vi "CANTest2.vi"() -> ()   [LabVIEW 2009]
uses:
  <vilib>/Platform/TimedLoop/XDataNode/XDataNode.xnode
  <vilib>/Platform/TimedLoop/XDataNode/loadlvalarms.vi
  <vilib>/Platform/TimedLoop/XDataNode/timing_clust.ctl
  <vilib>/Platform/TimedLoop/XDataNode/nitl_modes.ctl
  <vilib>/Platform/TimedLoop/XDataNode/wakeup.ctl
  <vilib>/Platform/TimedLoop/XDataNode/XDNodeRunTimeDep.lvlib
  CAN.lvlib
  Serial.lvlib
  CAN/SubVIs/CAN Jaguar Control Mode.ctl
panel:
  out "read buffer":u8[](array[numeric])
  out "is Timeout":bool
  out "is Corrupted":bool
  out "read data":u8[](array[numeric]) format="%.0x"
  in  "data":u8[](array[numeric]) format="%.0x"
  in  "messageID":u32 format="%.0x"
  out "error out":errorcluster
  in  "OK Button":bool
  in  "stop 2":bool
  in  "stop":bool
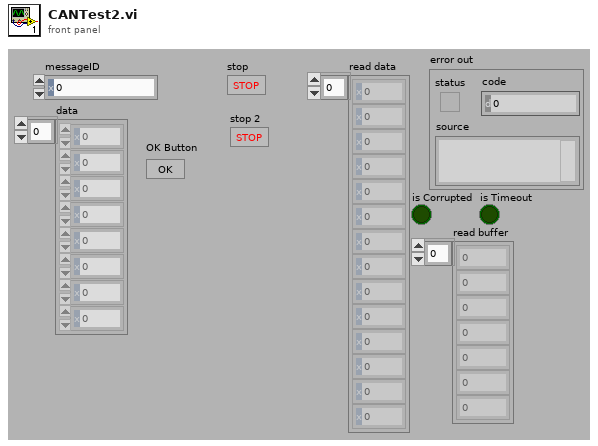
[diagram p1: front panel]
types:
  T1 = typedef "CAN.lvlib/CAN Jaguar Control Mode.ctl" = enum16{"Percent VBus", "Speed", "Position", "Current"}
  T2 = typedef "CAN.lvlib/CAN Jaguar Ref.ctl" = cluster{"Device Number":u8, "Control Mode":T1, "Inverted":bool, "Semaphore":T3, "Max Vout":dbl, "DevStatus":errorcluster}
  T3 = typedef "Semaphore RefNum" = refnum<k1>
  T4 = typedef "XDNodeRunTimeDep.lvlib/timing_clust.ctl" = cluster{"Expected End [f-1]":u64, "Actual End [f-1]":u64, "Finished Late? [f-1]":bool, "Expected End [i-1]":u64, "Actual End [i-1]":u64, "Finished Late? [i-1]":bool, "Expected Start [i]":u64, "Actual Start [i]":u64, "Expected Start [f]":u64, "Actual Start [f]":u64, "Source Name":string, "Structure Name":string, "Period":i64, "Deadline":i64, "Offset":i64, "Start":i64, "Priority":i32, "Timeout":i32, "Mode":T5, "Wakeup Reason":T6, "Error":errorcluster, "Source Type":string, "Secondary Source Type":string, "Global End Time":u64, "Global Start Time":u64, "Frame Duration":u64, "Iteration Duration":u64, "Assigned CPU":i32, "I/O Scan Engine Mode":u32}
  T5 = typedef "XDNodeRunTimeDep.lvlib/nitl_modes.ctl" = enum32{"No Change", "Process missed periods, maintain original phase", "Discard missed periods, maintain original phase", "Process missed periods, ignore original phase", "Discard missed periods, ignore original phase"}
  T6 = typedef "XDNodeRunTimeDep.lvlib/wakeup.ctl" = enum32{"Normal", "Aborted", "Asynchronous wakeup", "Timing source error", "Timed loop error", "Timeout"}
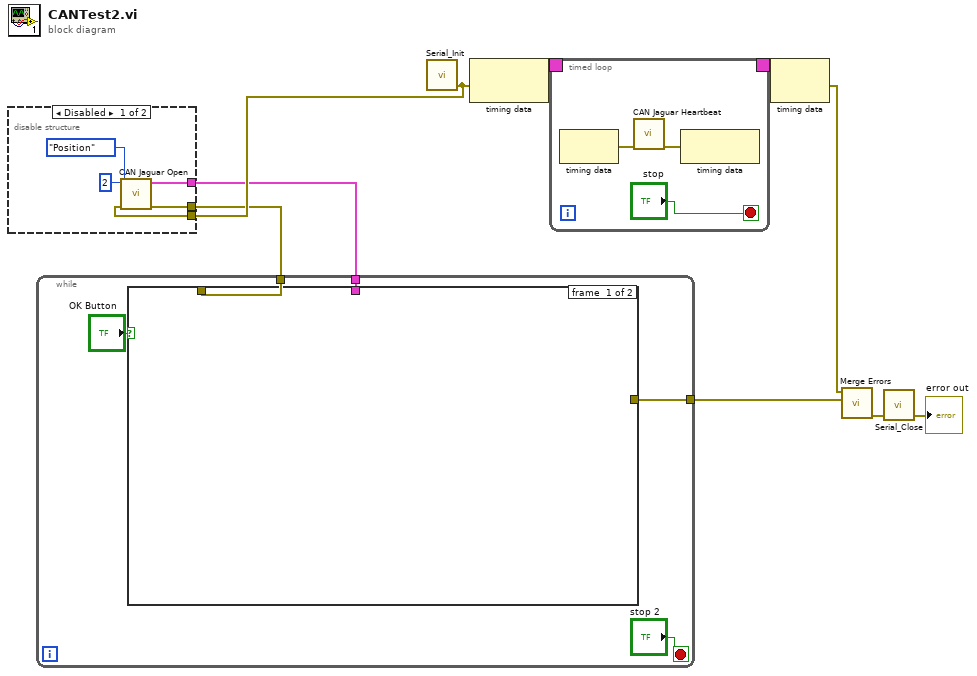
[diagram p0: block diagram]
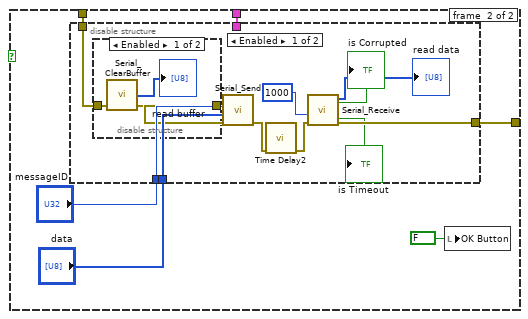
[diagram p3: hidden frame]
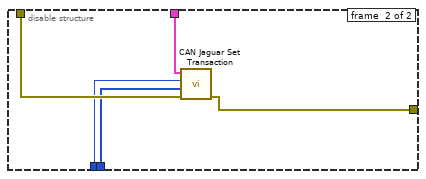
[diagram p5: hidden frame]
diagram:
  n1 = call "Serial_Init.vi"() -> ("error out"=w3:errorcluster)  [unwired: 4 in, 1 out]
  n2 = disable-structure shown="Disabled" {
    disable-tunnel: w3 -> [w12 _]
    disable-tunnel: [w11 _] -> w2
    disable-tunnel: [w10 _] -> w1
    frame #0 {
      n3 = call "CAN Jaguar Open.vi"("error in (no error)"=w12, "Control Mode"=CAN_Jaguar_Control_Mode."Position", "Device Number"=u8 2) -> ("error out"=w11:errorcluster, "CAN Jaguar Ref Out"=w10:T2)  [unwired: 7 in]
    }
    frame #1 {
    }
  }
  n4 = while {
    tunnel: [w18] -> w7
    tunnel: w2 -> [w16]
    tunnel: w1 -> [w15]
    stop <- "stop 2" stop-if-true
    n5 = case shown="True" "OK Button" {
      tunnel: [_ w23] -> w18
      tunnel: w16 -> [_ w21]
      tunnel: w15 -> [_ w20]
      frame #0 {
      }
      frame #1 {
        n6 = disable-structure shown="Enabled" {
          disable-tunnel: "messageID" -> [w36 w42]
          disable-tunnel: "data" -> [w35 w41]
          disable-tunnel: [w34 w44] -> w23
          disable-tunnel: w21 -> [w30 w45]
          disable-tunnel: w20 -> [_ w43]
          frame #0 {
            n7 = disable-structure shown="Enabled" {
              disable-tunnel: w30 -> [w39 w40]
              disable-tunnel: [w37 w40] -> w29
              frame #0 {
                n8 = call "Serial_ClearBuffer.vi"("error in (no error)"=w39) -> ("error out"=w37:errorcluster, "read data"=→"read buffer":u8[])  [unwired: 3 in]
              }
              frame #1 {
              }
            }
            n9 = call "Serial_Send.vi"("error in"=w29, "data"=w35, "messageID"=w36) -> ("error out"=w27:errorcluster)  [unwired: 7 in, 1 out]
            n10 = call "Time Delay2"("error in (no error)"=w27) -> ("error out"=w26:errorcluster)  [unwired: 10 in]
            n11 = call "Serial_Receive.vi"("error in (no error)"=w26, "timeoutMs"=u32 1000) -> ("error out"=w34:errorcluster, "read data"=→"read data":u8[], "is Timeout"=→"is Timeout":bool, "is Corrupted"=→"is Corrupted":bool)  [unwired: 4 in, 2 out]
          }
          frame #1 {
            n12 = call "CAN Jaguar Set Transaction.vi"("error in"=w45, "Data"=w41, "Message ID"=w42, "CAN Jaguar Ref"=w43) -> ("error out"=w44:errorcluster)  [unwired: 6 in, 1 out]
          }
        }
        n13 = local write "OK Button"(FALSE ("OK Button")) -> ()
      }
    }
  }
  n14 = node-c288(w3) -> (w9:T4)
  n15 = timed-loop {
    timing: w9 -> [_]
    timing-out: [_] -> w8
    stop <- "stop" stop-if-true
    n16 = node-c288() -> (w48:errorcluster)  [unwired: 1 in]
    n17 = call "CAN Jaguar Heartbeat.vi"("error in (no error)"=w48) -> ("error out"=w47:errorcluster)  [unwired: 10 in]
    n18 = node-c288(w47) -> ()  [unwired: 1 out]
  }
  n19 = node-c288(w8) -> (w6:errorcluster)
  n20 = call <vilib>:"Merge Errors.vi"("error in 2 (no error)"=w7, "error in 1 (no error)"=w6) -> ("error out"=w4:errorcluster)  [unwired: 5 in]
  n21 = call "Serial_Close.vi"("error in (no error)"=w4) -> ("error out"=→"error out":errorcluster)  [unwired: 4 in]
